vi "RT Driver VI.vi"(6 "Device Clock":string, 9 "Device Inputs FIFO":refnum<k33>, 10 "Device Outputs FIFO":refnum<k33>, 11 "Device Reference":T1 format="%.0x") -> ()   [LabVIEW 2017, in "NI-SWITCH Engine.lvlib"]
uses:
  NI-SWITCH Engine.lvlib
  <vilib>/NI Veristand/Custom Device API/Custom Device Item Ref.ctl
  <vilib>/NI Veristand/Custom Device API/Custom Device Channel Type.ctl
  Outputs With Indices.ctl
  Shared/FIFO Indices.ctl
  Includes/NISWITCHMessaging.lvlibp/NI-SWITCH Consumer/NI-SWITCH Consumer.lvclass
  C:/Dev/GitHub/niveristand-routing-and-faulting-custom-device/Includes/CDMessaging.lvlibp/Consumer/Abstract Consumer/Abstract Consumer.lvclass
  <vilib>/NI VeriStand/Custom Device API/Custom Device API.lvlib
  <vilib>/NI Veristand/Custom Device Tools/Custom Device Utility Library/Custom Device Utility Library.lvlib
  Includes/CDMessaging.lvlibp/Consumer/Abstract Consumer/Abstract Consumer.lvclass
  Shared/NI-SWITCH Shared.lvlib
panel:
  in  "Status Channel":dbl
  in  "Initialization Status Notifier":refnum<notifier>
  in  "Status Notifier":refnum<notifier>
  # "Custom Device Template\nv1.0"
  # "Use this template as a starting point for creating a custom device code module. The input controls shown here are specially named controls that the system will use to provide the device loop with data. The controls are not required for the device loop to run. For instance, if the device doesn't produce any output data, then you don't need the Device Outputs FIFO control. If you do use these controls, however, they need to have these exact names to be functional."
  # "The optional status notifier element is used to notify the RT engine of the last state of the custom device, and to indicate the device has completed execution. If this control is not used, a default No Error value is returned to the system when the device finishes execution.\n\nNote: This error state is not checked until the system shuts down. Use an output status channel to send more immediate status values to the system."
  # "This optional input can be used to send the VeriStand Engine the final status of the custom device initalization process. If this control exists on the custom device front panel, the VeriStand Engine will wait for a status update before starting up. If the custom device reports an error, that will abort the execution of the current configuration in the VeriStand Engine.\n\nThis control can be deleted if the custom device does not need to send the initialization status update."
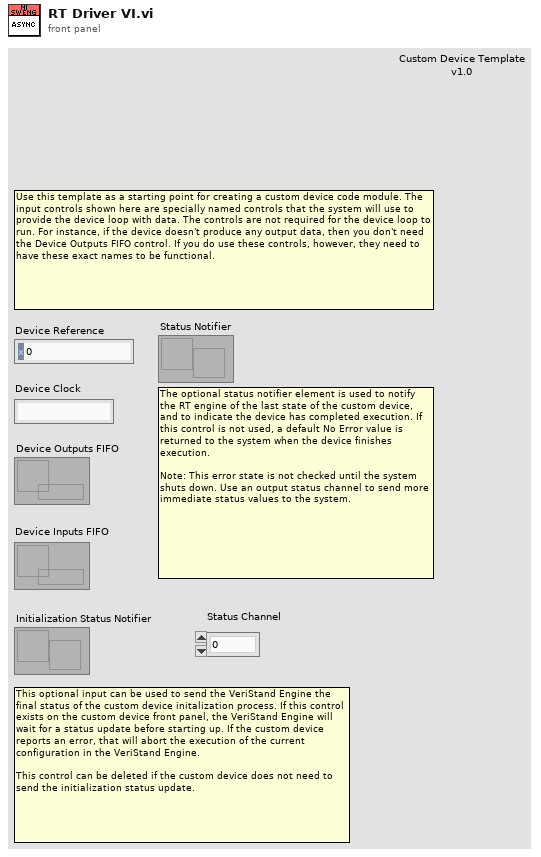
[diagram p1: front panel]
types:
  T1 = typedef "Custom Device API.lvlib/Custom Device Item Ref.ctl" = u64
  T2 = typedef "Custom Device API.lvlib/Custom Device Channel Type.ctl" = enum16{"Input", "Output"}
  T3 = typedef "NI-SWITCH Shared.lvlib/FIFO Indices.ctl" = cluster{"Status Channel":i32, "Heartbeat Channel":i32}
  T4 = typedef "Custom Device API.lvlib/Custom Device Engine Event Ref.ctl" = refnum<event-registration>
  T5 = typedef "NI-SWITCH Engine.lvlib/Outputs With Indices.ctl" = cluster{"Outputs":dbl[], "FIFO Indices":T3}
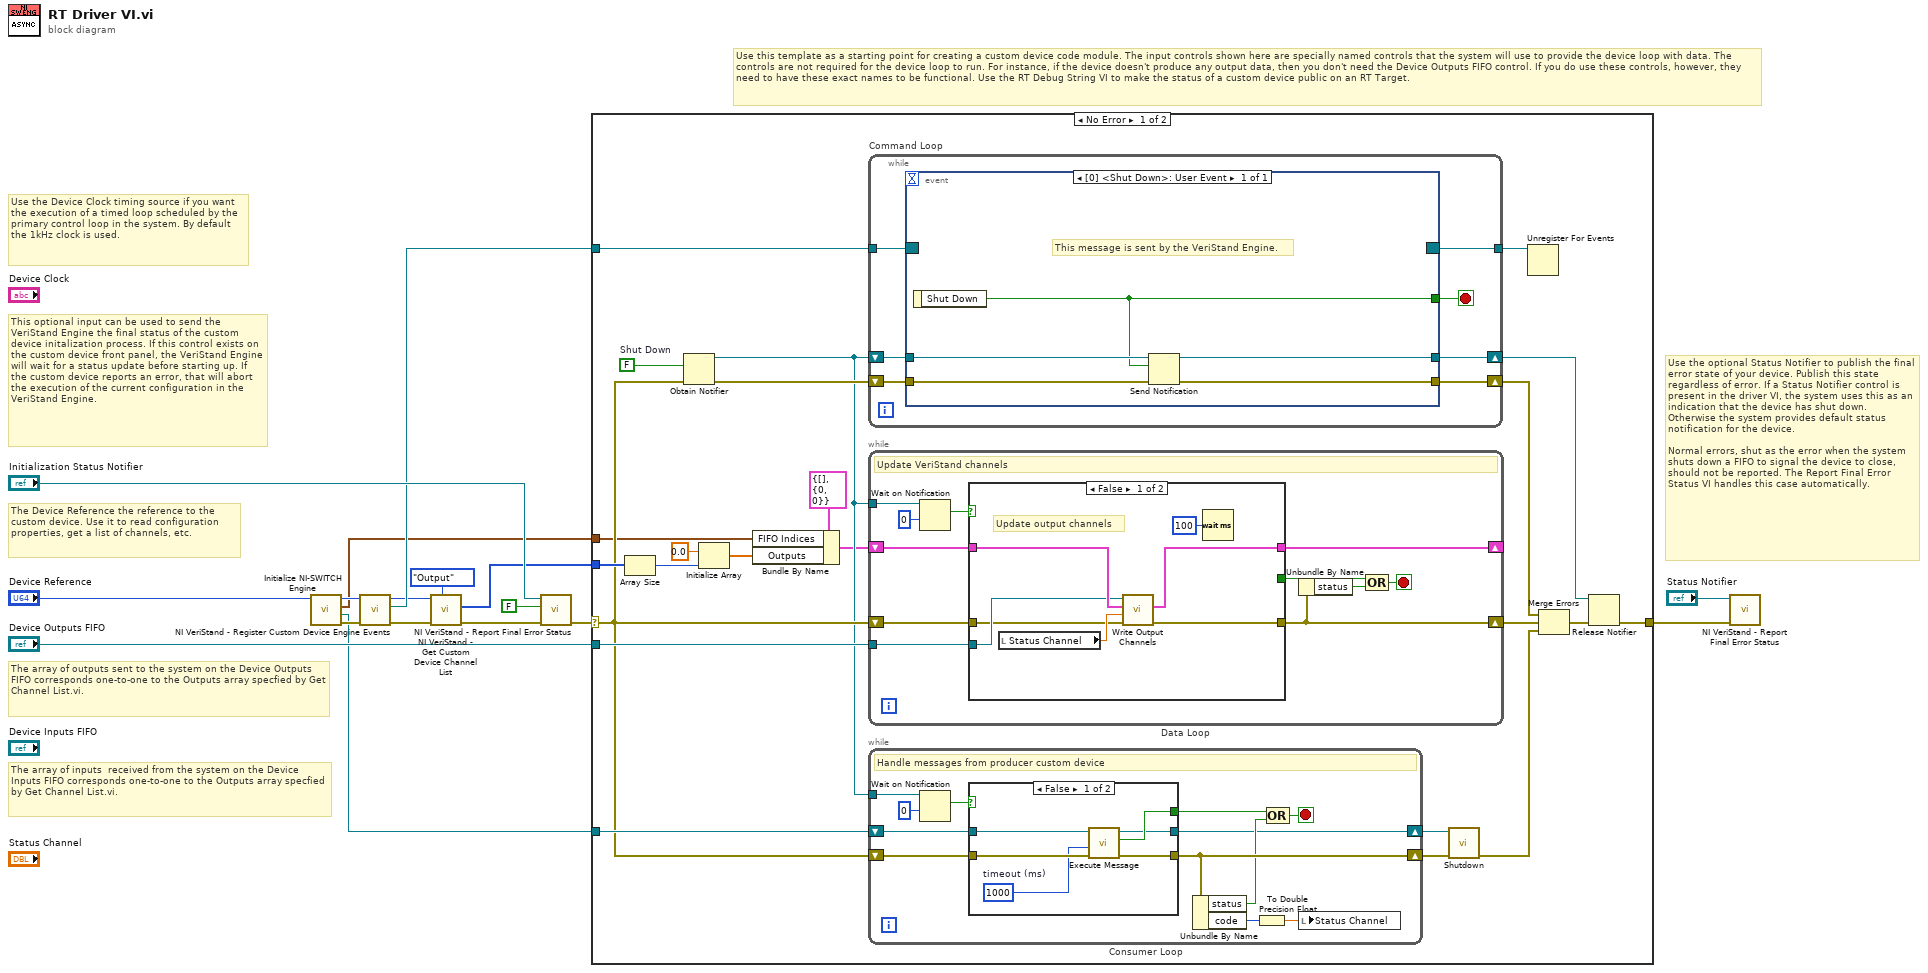
[diagram p0: block diagram]
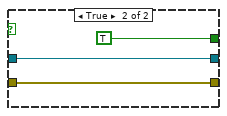
[diagram p2: hidden frame]
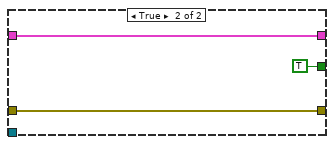
[diagram p3: hidden frame]
diagram:
  # "This optional input can be used to send the VeriStand Engine the final status of the custom device initalization process. If this control exists on the custom device front panel, the VeriStand Engine will wait for a status update before starting up. If the custom device reports an error, that will abort the execution of the current configuration in the VeriStand Engine."
  # "The array of inputs  received from the system on the Device Inputs FIFO corresponds one-to-one to the Outputs array specfied by Get Channel List.vi."
  # "Use the optional Status Notifier to publish the final error state of your device. Publish this state regardless of error. If a Status Notifier control is present in the driver VI, the system uses this as an indication that the device has shut down. Otherwise the system provides default status notification for the device.\n\nNormal errors, shut as the error when the system shuts down a FIFO to signal the device to close, should not be reported. The Report Final Error Status VI handles this case automatically."
  # "The array of outputs sent to the system on the Device Outputs FIFO corresponds one-to-one to the Outputs array specfied by Get Channel List.vi."
  # "The Device Reference the reference to the custom device. Use it to read configuration properties, get a list of channels, etc."
  # "Use the Device Clock timing source if you want the execution of a timed loop scheduled by the primary control loop in the system. By default the 1kHz clock is used."
  # "Use this template as a starting point for creating a custom device code module. The input controls shown here are specially named controls that the system will use to provide the device loop with data. The controls are not required for the device loop to run. For instance, if the device doesn't produce any output data, then you don't need the Device Outputs FIFO control. If you do use these controls, however, they need to have these exact names to be functional. Use the RT Debug String VI to make the status of a custom device public on an RT Target."
  n1 = call "Initialize NI-SWITCH Engine.vi"("Device Ref in"="Device Reference") -> ("error out"=w3:errorcluster, "NI-SWITCH Consumer"=w2:refnum<class "NI-SWITCH Consumer.lvclass">, "FIFO Indices"=w1:T3, "Device Ref out"=w4:T1)  [unwired: 7 in]
  n2 = call <vilib>:"NI VeriStand - Register Custom Device Engine Events.vi"("error in (no error)"=w3, "Device Ref in"=w4) -> ("error out"=w17:errorcluster, "Custom Device Engine Event Ref"=w10:T4, "Device Ref out"=w8:T1)  [unwired: 7 in]
  n3 = call <vilib>:"NI VeriStand - Get Custom Device Channel List.vi"("Channel Type"=Custom_Device_Channel_Type."Output", "error in (no error)"=w17, "Device Ref in"=w8) -> ("error out"=w13:errorcluster, "Specified Channel Ref List"=w12:T1[])  [unwired: 7 out]
  n4 = call <vilib>:"NI VeriStand - Report Final Error Status.vi"("error in (no error)"=w13, "Filter FIFO & Shutdown Errors (T)"=FALSE ("Filter FIFO Errors (T)"), "Status Notifier"="Initialization Status Notifier") -> ("error out"=w7:errorcluster)  [unwired: 8 out]
  n5 = case shown="No Error" w7 {
    selector: w7 -> [w26 w95]
    tunnel: "Device Outputs FIFO" -> [w39 _]
    tunnel: w12 -> [w36 _]
    tunnel: w10 -> [w35 _]
    tunnel: [w33 w95] -> w9
    tunnel: w2 -> [w27 _]
    tunnel: w1 -> [w23 _]
    frame No Error {
      w34 = FALSE  # Shut Down
      n6 = Array Size(array=w36) -> (size(s)=w37:i32)
      n7 = Obtain Notifier(notification data type=w34, error in (no error)=w26) -> (notifier out=w25:refnum<notifier>, error out=w40:errorcluster)  [unwired: 2 in, 1 out]
      n8 = Initialize Array(0.0 ("element"), w37) -> (w22:dbl[])
      n9 = Bundle By Name(cluster=T5 {"Outputs"=[], "FIFO Indices"={"Status Channel"=0, "Heartbeat Channel"=0}} ("Outputs"), "FIFO Indices"=w23, "Outputs"=w22) -> (w21:T5)
      n10 = while "Command Loop" {
        tunnel: w35 -> [w68]
        tunnel: [w67] -> w32
        shift-right: [w64] -> w31
        shift-left: w25 -> [w65]
        shift-right: [w62] -> w28
        shift-left: w40 -> [w63]
        stop <- w66 stop-if-true
        n11 = event shown="[0] <Shut Down>: User Event" {
          selector: w68 -> [_]
          dyn-events: [_] -> w67
          timeout: _ -> [_]
          tunnel: [w71] -> w66
          tunnel: w65 -> [w72]
          tunnel: [w73] -> w64
          tunnel: w63 -> [w70]
          tunnel: [w69] -> w62
          event User Event {
            # "This message is sent by the VeriStand Engine."
            n12 = event-data() -> ("Shut Down"=w71:bool)  [unwired: 1 in]
            n13 = Send Notification(notification=w71, notifier=w72, error in (no error)=w70) -> (notifier out=w73:refnum<notifier>, error out=w69:errorcluster)
          }
        }
      }
      n14 = while "Data Loop" {
        shift-right: [w79] -> w30
        shift-left: w26 -> [w84]
        shift-right: [w82] -> _
        shift-left: w21 -> [w83]
        tunnel: w39 -> [w81]
        tunnel: w25 -> [w78]
        stop <- w74 stop-if-true
        # "Update VeriStand channels"
        n15 = Wait on Notification(notifier=w78, timeout in ms (-1)=0) -> (notification=w77:bool)  [unwired: 2 in, 3 out]
        n16 = case shown="False" w77 {
          tunnel: w84 -> [w85 w94]
          tunnel: w83 -> [w90 w93]
          tunnel: [w88 w93] -> w82
          tunnel: w81 -> [w87 _]
          tunnel: [w89 w94] -> w79
          tunnel: [_ TRUE] -> w75
          frame False {
            # "Update output channels"
            n17 = local read "Status Channel"() -> (w86:dbl)
            n18 = call "Write Output Channels.vi"("error in (no error)"=w85, "Status"=w86, "Outputs"=w90, "Device Outputs FIFO"=w87) -> ("error out"=w89:errorcluster, "Updated Outputs"=w88:T5)  [unwired: 6 in]
            n19 = Wait (ms)(milliseconds to wait=u32 100) -> ()  [unwired: 1 out]
          }
          frame True {
          }
        }
        n20 = Unbundle By Name(w79) -> ("status"=w76:bool)
        n21 = Compound Arithmetic op=OR(w75, w76) -> (w74:bool)
      }
      n22 = while "Consumer Loop" {
        shift-right: [w48] -> w20
        shift-left: w26 -> [w49]
        tunnel: w25 -> [w46]
        shift-right: [w41] -> w18
        shift-left: w27 -> [w51]
        stop <- w52 stop-if-true
        # "Handle messages from producer custom device"
        n23 = Wait on Notification(notifier=w46, timeout in ms (-1)=0) -> (notification=w45:bool)  [unwired: 2 in, 3 out]
        n24 = case shown="False" w45 {
          tunnel: w51 -> [w58 w59]
          tunnel: [w57 TRUE ("Stop?")] -> w50
          tunnel: w49 -> [w56 w61]
          tunnel: [w55 w61] -> w48
          tunnel: [w54 w59] -> w41
          frame False {
            w53 = 1000  # timeout (ms)
            n25 = call "Execute Message.vi"("error in (no error)"=w56, "timeout in ms (-1)"=w53, "Abstract Consumer in"=w58) -> ("error out"=w55:errorcluster, "Stop?"=w57:bool, "Abstract Consumer out"=w54:refnum<class "Abstract Consumer.lvclass">)  [unwired: 5 in, 1 out]
          }
          frame True {
          }
        }
        n26 = Unbundle By Name(w48) -> ("status"=w44:bool, "code"=w43:i32)
        n27 = To Double Precision Float(number=w43) -> (double precision float=w42:dbl)
        n28 = Compound Arithmetic op=OR(w50, w44) -> (w52:bool)
        n29 = local write "Status Channel"(w42) -> ()
      }
      n30 = call "Shutdown.vi"("error in (no error)"=w20, "Abstract Consumer in"=w18) -> ("error out"=w19:errorcluster)  [unwired: 8 in, 1 out]
      n31 = Unregister For Events(event registration refnum=w32) -> ()  [unwired: 1 in, 1 out]
      n32 = Merge Errors(w28, w30, w19) -> (w29:errorcluster)
      n33 = Release Notifier(notifier=w31, error in (no error)=w29) -> (error out=w33:errorcluster)  [unwired: 1 in, 2 out]
    }
    frame Error {
    }
  }
  n34 = call <vilib>:"NI VeriStand - Report Final Error Status.vi"("error in (no error)"=w9, "Status Notifier"="Status Notifier") -> ()  [unwired: 1 in, 9 out]
